vi "trace_deinit.vi"() -> (1 "deInit seq.":string)   [LabVIEW 2021]
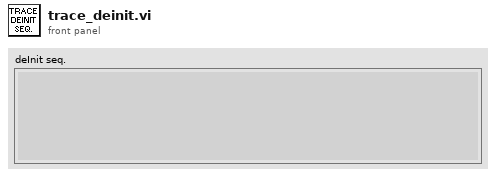
[diagram p1: front panel]
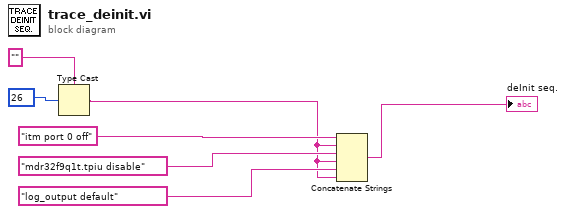
[diagram p0: block diagram]
diagram:
  n1 = Type Cast(type="", x=u8 26) -> (*(type *) &x=w1:string)
  n2 = Concatenate Strings("itm port 0 off" ("data in"), w1, "mdr32f9q1t.tpiu disable" ("data in"), w1, "log_output default" ("data in"), w1) -> (→"deInit seq.":string)
